vi "GUI.VISAResourceName.Get.vi"(8 "error in (no error)":errorcluster, 11 "deviceVISAName":string) -> (0 "error out":errorcluster, 2 "deviceVISAConnect":refnum<visa-resource-name>)   [LabVIEW 2019]
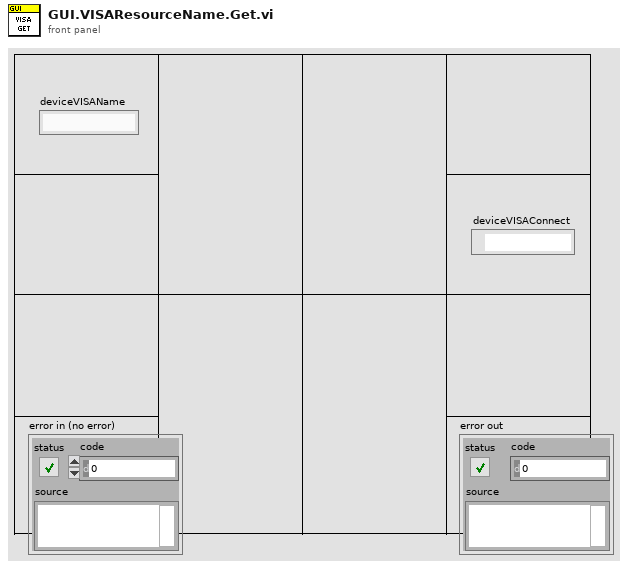
[diagram p1: front panel]
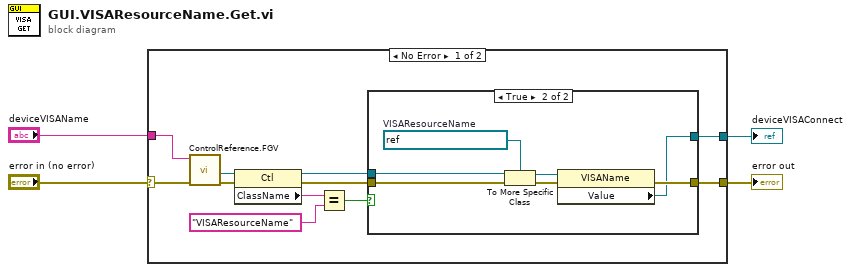
[diagram p0: block diagram]
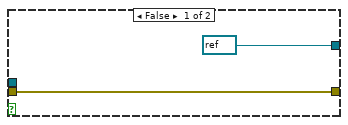
[diagram p2: hidden frame]
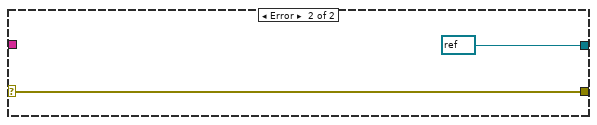
[diagram p3: hidden frame]
diagram:
  n1 = case shown="No Error" "error in (no error)" {
    selector: "error in (no error)" -> [w15 w26]
    tunnel: [w7 w26] -> w2
    tunnel: "deviceVISAName" -> [w6 _]
    tunnel: [w5 refnum<visa-resource-name> refnum ("Value")] -> w4
    frame No Error {
      n2 = call "ControlReference.FGV.vi"("error in (no error)"=w15, "controlLabelText"=w6) -> ("error out"=w13:errorcluster, "referenceToControl"=w14:refnum<vi>)  [unwired: 8 in]
      n3 = property class="Ctl"(reference=w14, error in=w13) -> (reference out=w9:refnum<vi>, error out=w8:errorcluster, "ClassName"=w12:string)
      n4 = Equal?(x=w12, y="VISAResourceName") -> (x = y?=w10:bool)
      n5 = case shown="True" w10 {
        tunnel: w9 -> [_ w23]
        tunnel: w8 -> [w17 w24]
        tunnel: [w17 w19] -> w7
        tunnel: [refnum<visa-resource-name> refnum ("Value") w18] -> w5
        frame False {
        }
        frame True {
          w22 = refnum<vi> refnum  # VISAResourceName
          n6 = To More Specific Class(target class=w22, reference=w23, error in=w24) -> (specific class reference=w21:refnum<vi>, error out=w20:errorcluster)
          n7 = property class="VISAName"(reference=w21, error in=w20) -> (error out=w19:errorcluster, "Value"=w18:refnum<visa-resource-name>)  [unwired: 1 out]
        }
      }
    }
    frame Error {
    }
  }
  "deviceVISAConnect" <- w4
  "error out" <- w2
